vi "MGI Bezier Inverse Old.vi"(1 "y":sgl format="%.2f", 2 "First k":i32, 3 "Bezier Control Points[]":sgl[](array[numeric]) format="%.4f") -> (0 "u":sgl format="%.2f")   [LabVIEW 2016]
doc: "Calculate a bezier 0..1 parameter from y, a bezier function result.\n\nAuthored by David A. Moore\nsupport@mooregoodideas.com\nwww.mooregoodideas.com\n\nCopyright (c) 2010, Moore Good Ideas, Inc.\n\nAll rights reserved.\n\nRedistribution and use in source and binary forms, with or without modification, are permitted provided that the following conditions are met:\n\n * Redistributions of source code must retain the above copyright notice, this list of conditions and the following disclaimer.\n * Redistributions in binary form must reproduce the above copyright notice, this list of conditions and the following disclaimer in the documentation and/or other materials provided with the distribution.\n * Neither the name of Moore Good Ideas, Inc. nor the names of its contributors may be used to endorse or promote products derived from this software without specific prior written permission.\n\nTHIS SOFTWARE IS PROVIDED BY THE COPYRIGHT HOLDERS AND CONTRIBUTORS \"AS IS\" AND ANY EXPRESS OR IMPLIED WARRANTIES, INCLUDING, BUT NOT LIMITED TO, THE IMPLIED WARRANTIES OF MERCHANTABILITY AND FITNESS FOR A PARTICULAR PURPOSE ARE DISCLAIMED. IN NO EVENT SHALL THE COPYRIGHT OWNER OR CONTRIBUTORS BE LIABLE FOR ANY DIRECT, INDIRECT, INCIDENTAL, SPECIAL, EXEMPLARY, OR CONSEQUENTIAL DAMAGES (INCLUDING, BUT NOT LIMITED TO, PROCUREMENT OF SUBSTITUTE GOODS OR SERVICES; LOSS OF USE, DATA, OR PROFITS; OR BUSINESS INTERRUPTION) HOWEVER CAUSED AND ON ANY THEORY OF LIABILITY, WHETHER IN CONTRACT, STRICT LIABILITY, OR TORT (INCLUDING NEGLIGENCE OR OTHERWISE) ARISING IN ANY WAY OUT OF THE USE OF THIS SOFTWARE, EVEN IF ADVISED OF THE POSSIBILITY OF SUCH DAMAGE.i"
panel:
  # "k"
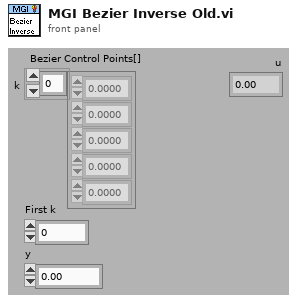
[diagram p1: front panel]
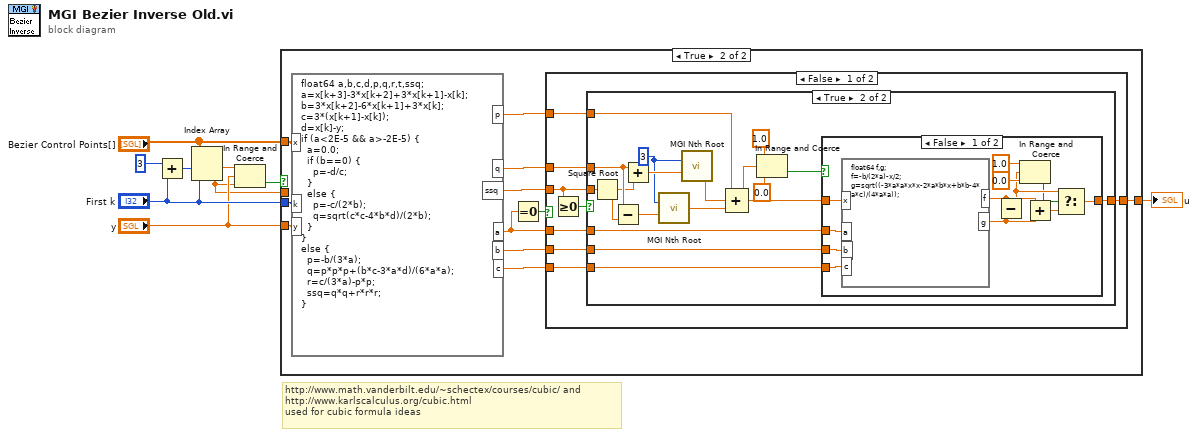
[diagram p0: block diagram]
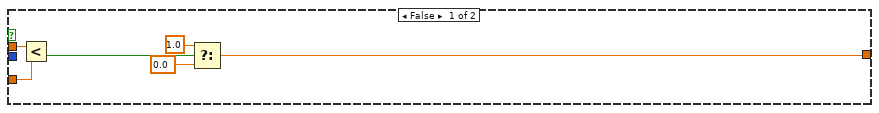
[diagram p2: hidden frame]
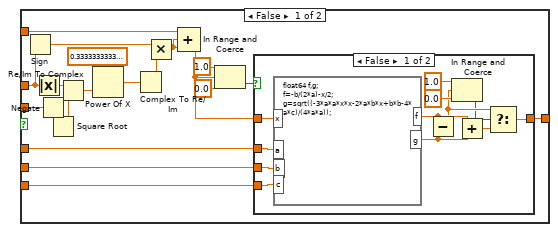
[diagram p3: hidden frame]
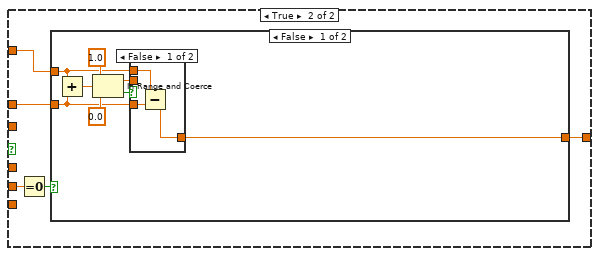
[diagram p6: hidden frame]
diagram:
  # "http://www.math.vanderbilt.edu/~schectex/courses/cubic/ and\nhttp://www.karlscalculus.org/cubic.html\nused for cubic formula ideas"
  n1 = Add(x=3, y="First k") -> (x+y=w9:i32)
  n2 = Index Array(array="Bezier Control Points[]", index #1=w9, index #2="First k") -> (element #1=w4:sgl, element #2=w1:sgl)
  n3 = In Range and Coerce(upper limit=w4, x="y", lower limit=w1) -> (In Range?=w2:bool)  [unwired: 1 out]
  n4 = case shown="True" w2 {
    tunnel: [w13 w23] -> w5
    tunnel: "First k" -> [_ w18]
    tunnel: "Bezier Control Points[]" -> [_ w17]
    tunnel: "y" -> [w11 w16]
    tunnel: w1 -> [w12 _]
    frame False {
      n5 = Less?(x=w12, y=w11) -> (x < y?=w10:bool)
      n6 = Select(t=1.0, s=w10, f=0.0) -> (s? t:f=w13:dbl)
    }
    frame True {
      n7 = formula code="float64 a,b,c,d,p,q,r,t,ssq;\na=x[k+3]-3*x[k+2]+3*x[k+1]-x[k];\nb=3*x[k+2]-6*x[k+1]+3*x[k];\nc=3*(x[k+1]-x[k]);\nd=x[k]-y;\nif (a<2E-5 && a>-2E-5) {\n  a=0.0;\n  if (b==0) {\n    p=-d/c;\n  }\n  else {\n    p=-c/(2*b);\n    q=sqrt(c*c-4*b*d)/(2*b);\n  }\n}\nelse {\n  p=-b/(3*a);\n  q=p*p*p+(b*c-3*a*d)/(6*a*a);\n  r=c/(3*a)-p*p;\n  ssq=q*q+r*r*r;\n}"("x"=w17, "y"=w16, "k"=w18) -> ("p"=w24:dbl, "q"=w26:dbl, "ssq"=w25:dbl, "a"=w20:dbl, "b"=w21:dbl, "c"=w19:dbl)
      n8 = Equal To 0?(x=w20) -> (x = 0?=w22:bool)
      n9 = case shown="False" w22 {
        tunnel: w26 -> [w34 w101]
        tunnel: w25 -> [w31 _]
        tunnel: w24 -> [w33 w100]
        tunnel: [w32 w102] -> w23
        tunnel: w21 -> [w28 w99]
        tunnel: w20 -> [w29 _]
        tunnel: w19 -> [w27 _]
        frame False {
          n10 = Greater Or Equal To 0?(x=w31) -> (x >= 0?=w30:bool)
          n11 = case shown="True" w30 {
            tunnel: w34 -> [w45 w84]
            tunnel: w33 -> [w49 w77]
            tunnel: [w36 w71] -> w32
            tunnel: w31 -> [w54 w76]
            tunnel: w29 -> [w39 w70]
            tunnel: w28 -> [w38 w69]
            tunnel: w27 -> [w37 w68]
            frame False {
              n12 = Sign(1:w45) -> (0:w44:dbl)
              n13 = Absolute Value(x=w45) -> (abs(x)=w46:dbl)
              n14 = Negate(x=w54) -> (-x=w53:dbl)
              n15 = Square Root(x=w53) -> (sqrt(x)=w52:dbl)
              n16 = Re/Im To Complex(1:w52, 2:w46) -> (0:w51:cdb)
              n17 = Power Of X(1:w51, 2:cdb 0.3333333333333333-0.0i ("1/x")) -> (0:w50:cdb)
              n18 = Complex To Re/Im(x + iy=w50) -> (x=w43:dbl)  [unwired: 1 out]
              n19 = Multiply(x=w44, y=w43) -> (x*y=w42:dbl)
              n20 = Compound Arithmetic op=ADD(w49, w42, w42) -> (w40:dbl)
              n21 = In Range and Coerce(upper limit=1.0, x=w40, lower limit=0.0) -> (In Range?=w41:bool)  [unwired: 1 out]
              n22 = case shown="False" w41 {
                tunnel: w40 -> [w66 w67]
                tunnel: [w55 w67] -> w36
                tunnel: w39 -> [w65 _]
                tunnel: w38 -> [w64 _]
                tunnel: w37 -> [w63 _]
                frame False {
                  n23 = formula code="float64 f,g;\nf=-b/(2*a)-x/2;\ng=sqrt((-3*a*a*x*x-2*a*b*x+b*b-4*a*c)/(4*a*a));"("x"=w66, "a"=w65, "b"=w64, "c"=w63) -> ("f"=w60:dbl, "g"=w59:dbl)
                  n24 = Subtract(x=w60, y=w59) -> (x-y=w57:dbl)
                  n25 = In Range and Coerce(upper limit=1.0, x=w57, lower limit=0.0) -> (In Range?=w56:bool)  [unwired: 1 out]
                  n26 = Add(x=w60, y=w59) -> (x+y=w58:dbl)
                  n27 = Select(t=w57, s=w56, f=w58) -> (s? t:f=w55:dbl)
                }
                frame True {
                }
              }
            }
            frame True {
              w80 = 3 ("Root")
              n28 = Square Root(x=w76) -> (sqrt(x)=w83:dbl)
              n29 = Subtract(x=w84, y=w83) -> (x-y=w81:dbl)
              n30 = Add(x=w84, y=w83) -> (x+y=w82:dbl)
              n31 = call <userlib>:"MGI Nth Root.vi"("Root"=w80, "x"=w81) -> ("Numeric"=w79:dbl)  [unwired: 13 in]
              n32 = call <userlib>:"MGI Nth Root.vi"("Root"=w80, "x"=w82) -> ("Numeric"=w78:dbl)  [unwired: 13 in]
              n33 = Compound Arithmetic op=ADD(w77, w78, w79) -> (w73:dbl)
              n34 = In Range and Coerce(upper limit=1.0, x=w73, lower limit=0.0) -> (In Range?=w72:bool)  [unwired: 1 out]
              n35 = case shown="False" w72 {
                tunnel: w73 -> [w96 w97]
                tunnel: [w85 w97] -> w71
                tunnel: w70 -> [w95 _]
                tunnel: w69 -> [w94 _]
                tunnel: w68 -> [w93 _]
                frame False {
                  n36 = formula code="float64 f,g;\nf=-b/(2*a)-x/2;\ng=sqrt((-3*a*a*x*x-2*a*b*x+b*b-4*a*c)/(4*a*a));"("x"=w96, "a"=w95, "b"=w94, "c"=w93) -> ("f"=w90:dbl, "g"=w89:dbl)
                  n37 = Subtract(x=w90, y=w89) -> (x-y=w87:dbl)
                  n38 = In Range and Coerce(upper limit=1.0, x=w87, lower limit=0.0) -> (In Range?=w86:bool)  [unwired: 1 out]
                  n39 = Add(x=w90, y=w89) -> (x+y=w88:dbl)
                  n40 = Select(t=w87, s=w86, f=w88) -> (s? t:f=w85:dbl)
                }
                frame True {
                }
              }
            }
          }
        }
        frame True {
          n41 = Equal To 0?(x=w99) -> (x = 0?=w98:bool)
          n42 = case shown="False" w98 {
            tunnel: [w105 w115] -> w102
            tunnel: w101 -> [w104 _]
            tunnel: w100 -> [w103 w115]
            frame False {
              n43 = Add(x=w103, y=w104) -> (x+y=w110:dbl)
              n44 = In Range and Coerce(upper limit=1.0, x=w110, lower limit=0.0) -> (coerced(x)=w106:dbl, In Range?=w107:bool)
              n45 = case shown="False" w107 {
                tunnel: w106 -> [_ w114]
                tunnel: [w111 w114] -> w105
                tunnel: w104 -> [w113 _]
                tunnel: w103 -> [w112 _]
                frame False {
                  n46 = Subtract(x=w112, y=w113) -> (x-y=w111:dbl)
                }
                frame True {
                }
              }
            }
            frame True {
            }
          }
        }
      }
    }
  }
  "u" <- w5
